vi "Power Supply Control Panel (No Objects).vi"(8 "error in (no error)":errorcluster) -> (0 "error out":errorcluster)   [LabVIEW 2012]
uses:
  Magnet status.ctl
  Oxford/PSSUBS.LLB/PSIO.ctl
  Oxford/BUSGEN.LLB/OxfordAddress.ctl
  Power Supply.lvclass
panel:
  in  "tada":string="Sound\\XP Sounds\\tada.wav"
  out "*ips120 (No Ob)":T4={"Field"=0.0, "Rate"=0.0, "Status"={"Sweeping"=FALSE, "Clamped"=FALSE, "Hold"=FALSE, "At Rest"=FALSE, "Quench"=FALSE, "Persistent Mode"=FALSE, "Switch Heater"=FALSE}, "ILM Shut Down?"=FALSE, "IO Info"={"Address"={"Com Port"=1, "ISOBUS Address"=2, "GPIB Address"=24, "Communication"=enum."ISOBUS"}, "Version"=enum."IPS"}, "IO Info (Level Meter)"={"Address"={"Com Port"=1, "ISOBUS Address"=5, "GPIB Address"=24, "Communication"=enum."ISOBUS"}, "ILM Name"="", "Display Channel"=[]}, "Training?"=FALSE, "Training Field and Speed Cluster"={"Training Field"=[0.0, 4.108, 5.78, 8.001], "Training Speed"=[0.0057, 0.0022833333333333334, 0.0011333333333333334, 0.0011333333333333334]}}
  in  "Cluster In":T4={"Field"=0.0, "Rate"=0.0, "Status"={"Sweeping"=FALSE, "Clamped"=FALSE, "Hold"=FALSE, "At Rest"=FALSE, "Quench"=FALSE, "Persistent Mode"=FALSE, "Switch Heater"=FALSE}, "ILM Shut Down?"=FALSE, "IO Info"={"Address"={"Com Port"=1, "ISOBUS Address"=2, "GPIB Address"=24, "Communication"=enum."ISOBUS"}, "Version"=enum."IPS"}, "IO Info (Level Meter)"={"Address"={"Com Port"=1, "ISOBUS Address"=5, "GPIB Address"=24, "Communication"=enum."ISOBUS"}, "ILM Name"="", "Display Channel"=[]}, "Training?"=FALSE, "Training Field and Speed Cluster"={"Training Field"=[0.0, 4.108, 5.78, 8.001], "Training Speed"=[0.0057, 0.0022833333333333334, 0.0011333333333333334, 0.0011333333333333334]}}
  out "Was at persistent?":bool
  in  "Return to persistent?":bool
  out "log counter":dbl
  out "Going to Field?":bool
  out "Current Field":dbl[unit]
  out "Update UI":bool
  out "Status":T1
  in  "Abort Field Sweep":bool
  out "done?":bool
  out "ILM Shut Down?":bool
  out "SH On":bool caption="Switch Heater"
  out "Persistent Mode":bool
  in  "SHcontrol":bool caption="Switch Heater"
  in  "gotopersistent":bool
  out "active":bool
  in  "Train\nMagnet":bool
  out "Busy":bool
  out "ready?":bool
  in  "rate":dbl[unit]=0.016666666666666666 caption="Rate" min=0.0 max=0.25
  in  "Goto":dbl[unit]
  in  "Clamp":bool
  in  "Check for Magnet":bool
  in  "Hold":bool
  in  "Goto Zero":bool
  in  "Goto Field":bool
  in  "endprgm":bool
  # "Magnet Control Panel"
  # "(at current field)"
  # "Off"
  # "On"
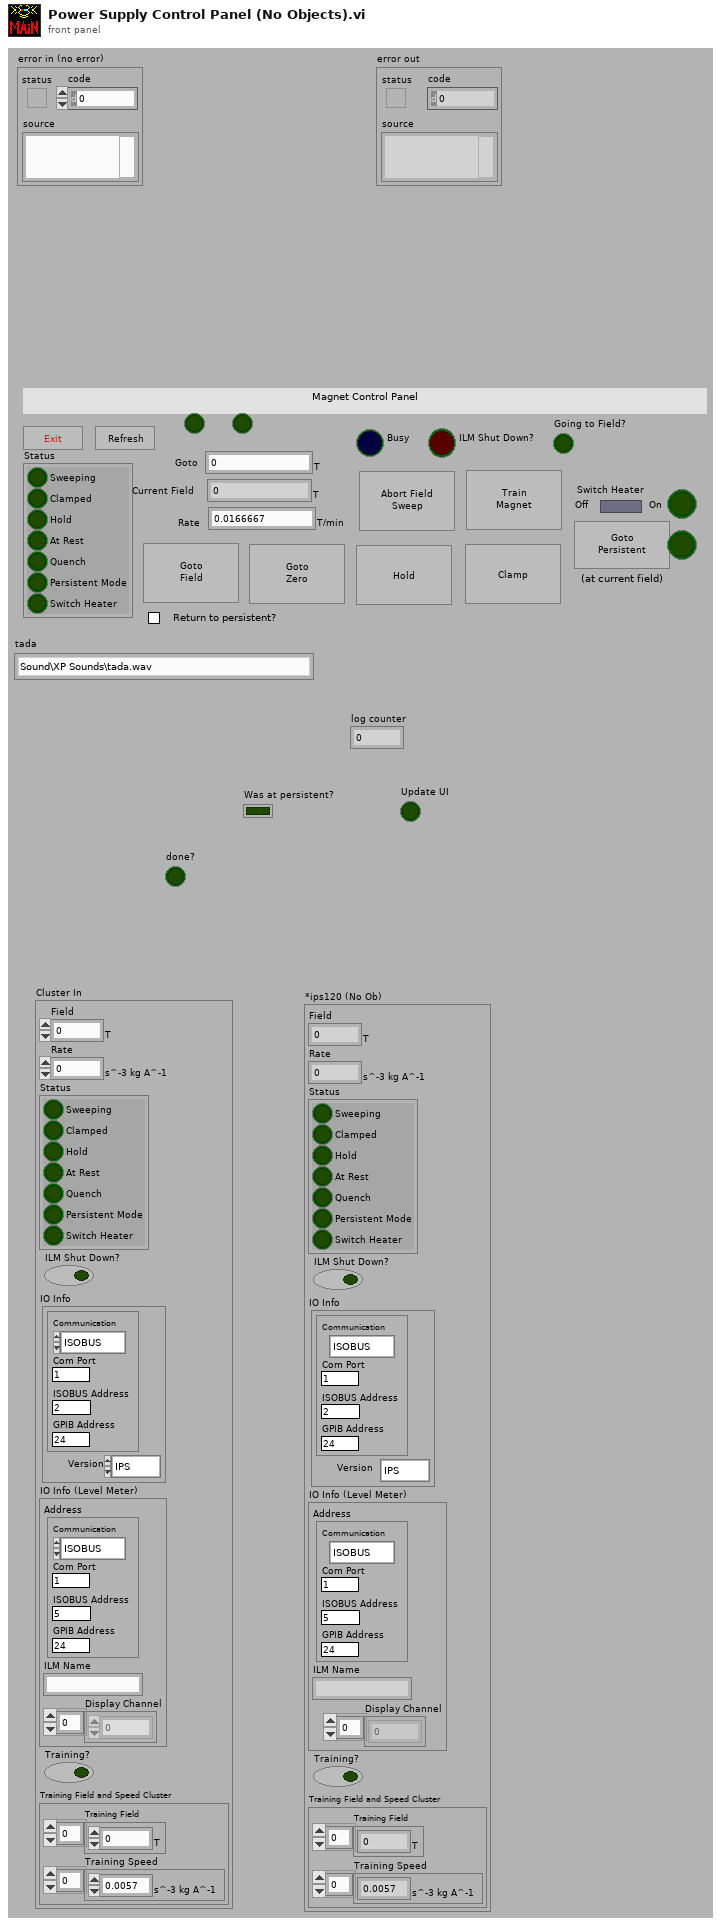
[diagram p1: front panel]
types:
  T1 = typedef "Power Supply.lvclass/Magnet status.ctl" = cluster{"Sweeping":bool, "Clamped":bool, "Hold":bool, "At Rest":bool, "Quench":bool, "Persistent Mode":bool, "Switch Heater":bool}
  T2 = typedef "PSIO.ctl" = cluster{"Address":T3, "Version":enum16{"PS", "IPS"}}
  T3 = typedef "OxfordAddress.ctl" = cluster{"Com Port":i32, "ISOBUS Address":i32, "GPIB Address":i16, "Communication":enum16{"RS232", "ISOBUS", "GPIB", "Gateway"}}
  T4 = cluster{"Field":dbl[unit], "Rate":dbl[unit], "Status":T1, "ILM Shut Down?":bool, "IO Info":T2, "IO Info (Level Meter)":cluster{"Address":T3, "ILM Name":string, "Display Channel":i32[]}, "Training?":bool, "Training Field and Speed Cluster":cluster{"Training Field":dbl[unit][], "Training Speed":dbl[unit][]}}
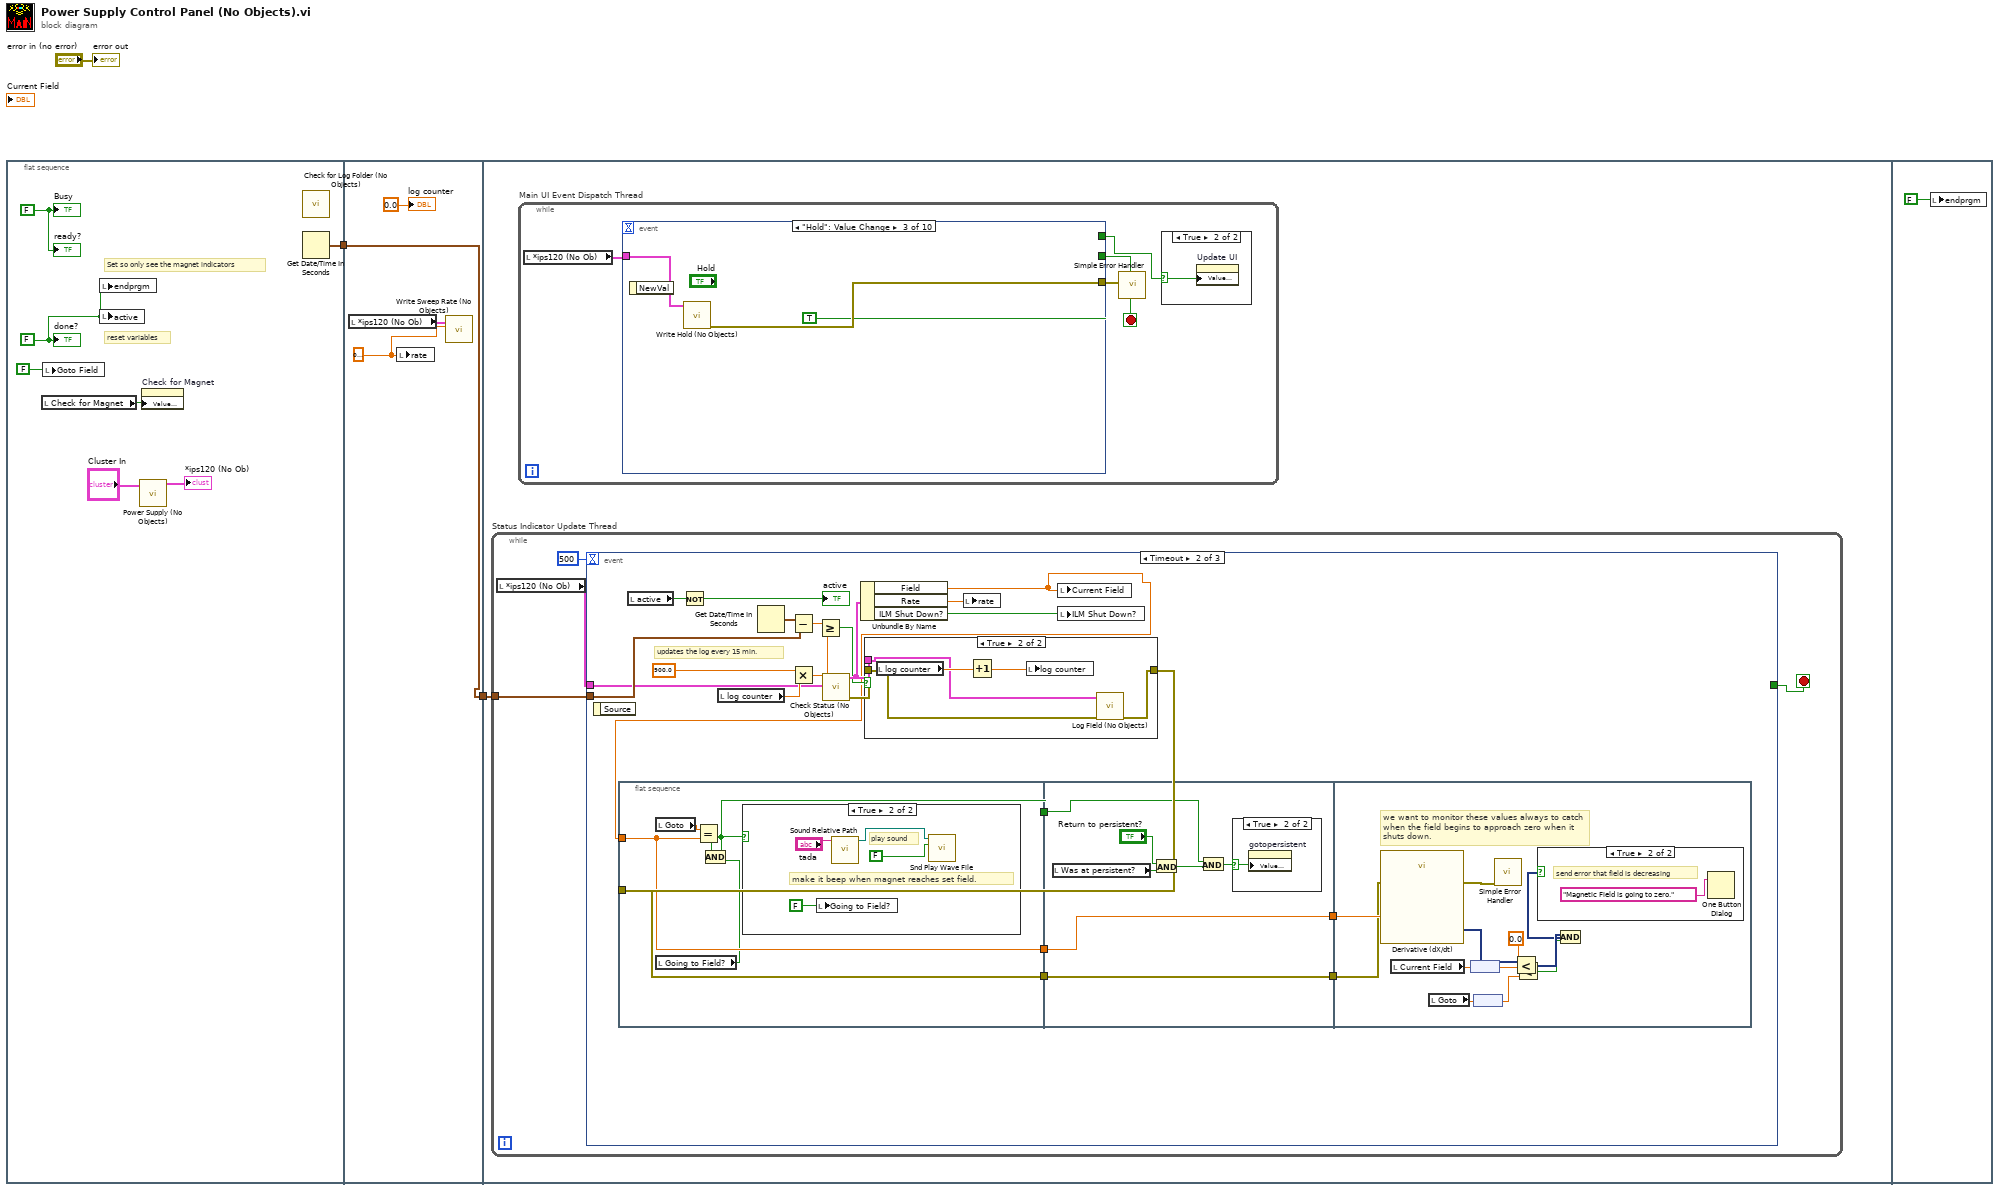
[diagram p0: block diagram]
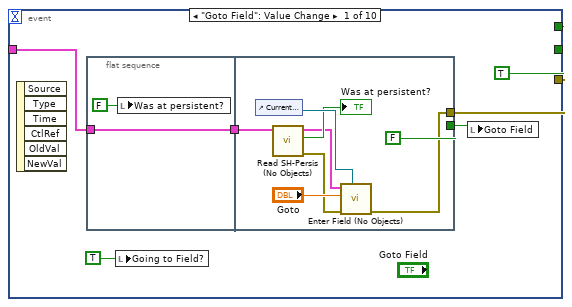
[diagram p3: hidden frame]
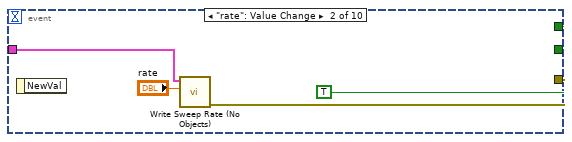
[diagram p4: hidden frame]
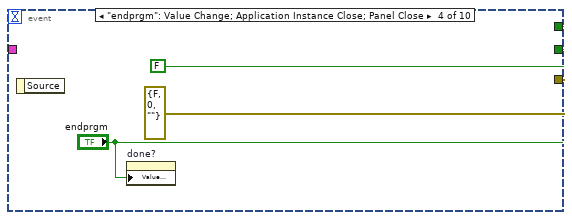
[diagram p5: hidden frame]
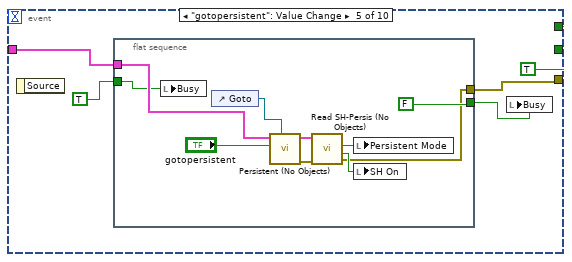
[diagram p6: hidden frame]
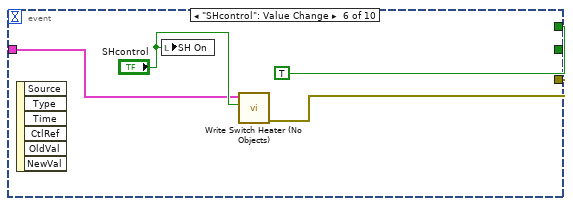
[diagram p7: hidden frame]
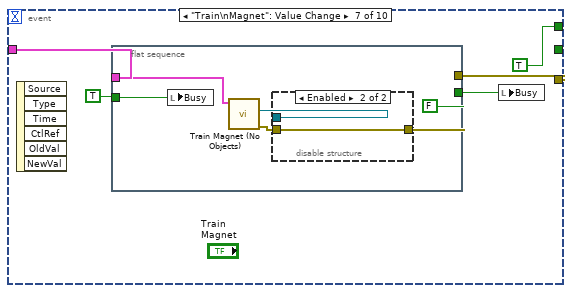
[diagram p8: hidden frame]
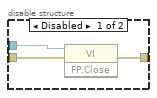
[diagram p9: hidden frame]
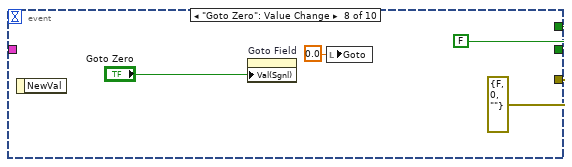
[diagram p10: hidden frame]
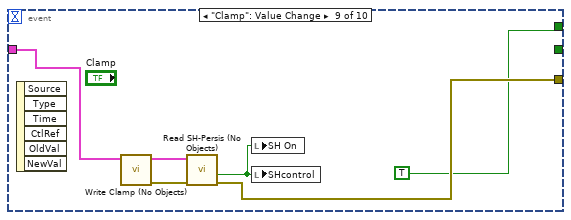
[diagram p11: hidden frame]
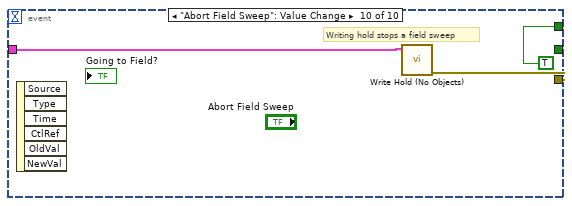
[diagram p12: hidden frame]
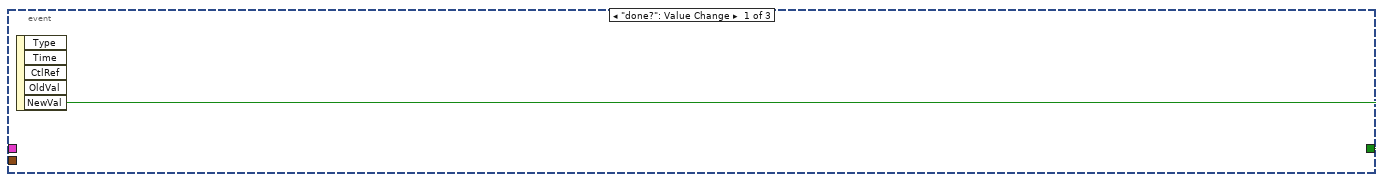
[diagram p13: hidden frame]
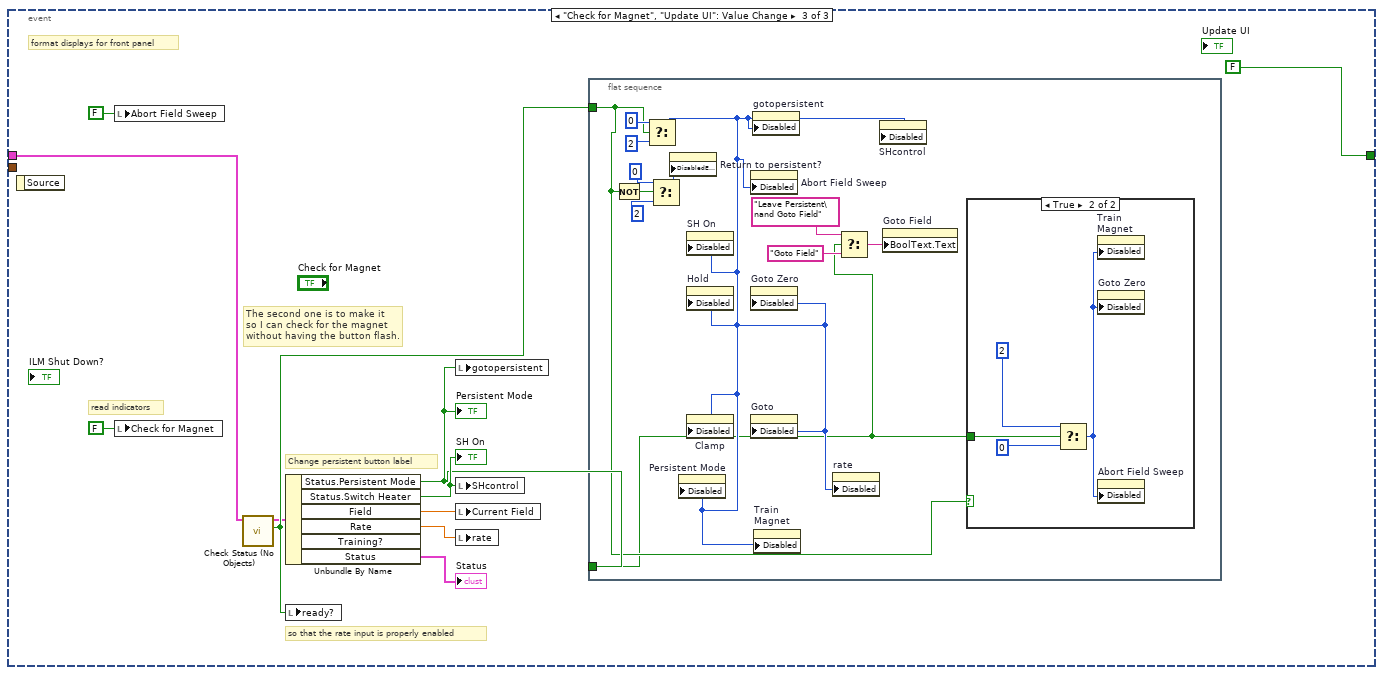
[diagram p18: hidden frame]
diagram:
  n1 = flat-sequence {
    tunnel: [w6] -> w2
    tunnel: w2 -> [w11]
    tunnel: [w11] -> w1
    tunnel: w1 -> [w15]
    frame #0 {
      w10 = FALSE
      w8 = FALSE
      # "Set so only see the magnet indicators"
      # "reset variables"
      n2 = local read "Check for Magnet"() -> (w9:bool)
      n3 = local write "Goto Field"(FALSE ("active")) -> ()
      n4 = local write "endprgm"(w8) -> ()
      n5 = local write "active"(w8) -> ()
      n6 = call "Power Supply (No Objects).vi"("Cluster In"="Cluster In") -> ("Cluster Out"=→"*ips120 (No Ob)":T4)  [unwired: 9 in, 1 out]
      n7 = property on="Check for Magnet" class="Bool (strict)"("Value (Signaling)"=w9) -> ()  [unwired: 2 in, 2 out]
      n8 = call "Check for Log Folder (No Objects).vi"() -> ()  [unwired: 1 in]
      n9 = Get Date/Time In Seconds() -> (seconds since 1Jan1904=w6:timestamp)
      "ready?" <- w10
      "Busy" <- w10
      "done?" <- w8
    }
    frame #1 {
      w12 = dbl[unit] 0.016666666666666666 ("rate")
      n10 = local read "*ips120 (No Ob)"() -> (w13:T4)
      n11 = local write "rate"(w12) -> ()
      n12 = call "Write Sweep Rate (No Objects).vi"("rate"=w12, "Cluster In"=w13) -> ()  [unwired: 8 in, 2 out]
      "log counter" <- 0.0 ("log counter")
    }
    frame #2 {
      n13 = while "Status Indicator Update Thread" {
        tunnel: w15 -> [w96]
        stop <- w94 stop-if-true
        n14 = local read "*ips120 (No Ob)"() -> (w95:T4)
        n15 = event shown="[1] Timeout" {
          selector: _ -> [_ _ _]
          dyn-events: _ -> [_ _ _]
          timeout: 500 -> [_ _ _]
          tunnel: [w98 _ FALSE] -> w94
          tunnel: w95 -> [_ w101 w158]
          tunnel: w96 -> [_ w117 _]
          event "done?": Value Change {
            n16 = event-data() -> ("NewVal"=w98:bool)  [unwired: 5 out]
          }
          event Timeout {
            # "updates the log every 15 min."
            n17 = event-data() -> ()  [unwired: 2 out]
            n18 = flat-sequence {
              tunnel: w100 -> [w125]
              tunnel: w99 -> [w123]
              tunnel: [w123] -> w106
              tunnel: [w125] -> w105
              tunnel: [w120] -> w104
              tunnel: w106 -> [w136]
              tunnel: [w136] -> w103
              tunnel: w105 -> [w135]
              tunnel: [w135] -> w102
              tunnel: w104 -> [w133]
              tunnel: w103 -> [w149]
              tunnel: w102 -> [w148]
              frame #0 {
                n19 = local read "Goto"() -> (w124:dbl[unit])
                n20 = local read "Going to Field?"() -> (w121:bool)
                n21 = Equal?(x=w124, y=w123) -> (x = y?=w122:bool)
                n22 = And(x=w122, y=w121) -> (x .and. y?=w120:bool)
                n23 = case shown="True" w120 {
                  frame False {
                  }
                  frame True {
                    # "make it beep when magnet reaches set field."
                    # "play sound"
                    n24 = local write "Going to Field?"(FALSE ("Going to Field?")) -> ()
                    n25 = call "Sound Relative Path.vi"("Sound"="tada") -> ("Relative Path"=w128:path)  [unwired: 10 in]
                    n26 = call <vilib>:"Snd Play Wave File.vi"("wait until finish (T)"=FALSE, "wave file path"=w128) -> ()  [unwired: 1 in, 9 out]
                  }
                }
              }
              frame #1 {
                n27 = local read "Was at persistent?"() -> (w132:bool)
                n28 = And(x="Return to persistent?", y=w132) -> (x .and. y?=w130:bool)
                n29 = And(x=w133, y=w130) -> (x .and. y?=w134:bool)
                n30 = case shown="True" w134 {
                  selector: w134 -> [_ w137]
                  frame False {
                  }
                  frame True {
                    n31 = property on="gotopersistent" class="Bool (strict)"("Value (Signaling)"=w137) -> ()  [unwired: 2 in, 2 out]
                  }
                }
              }
              frame #2 {
                # "we want to monitor these values always to catch\nwhen the field begins to approach zero when it\nshuts down."
                n32 = call "Derivative (dX/dt)"("error in (no error)"=w148, "Signals"=w149) -> ("error out"=w143:errorcluster, "Result"=w147:dynamicdata)  [unwired: 4 out]
                n33 = local read "Current Field"() -> (w139:dbl[unit])
                n34 = local read "Goto"() -> (w141:dbl[unit])
                n35 = node(w139) -> (w138:dbl)
                n36 = node(w141) -> (w140:dbl)
                n37 = call <vilib>:"Simple Error Handler.vi"("error in (no error)"=w143) -> ()  [unwired: 4 in, 5 out]
                n38 = Less?(x=w147, y=0.0) -> (x < y?=w145:dynamicdata)
                n39 = Less?(x=w138, y=w140) -> (x < y?=w142:bool)
                n40 = And(x=w145, y=w142) -> (x .and. y?=w144:dynamicdata)
                n41 = case shown="True" w144 {
                  frame False {
                  }
                  frame True {
                    # "send error that field is decreasing"
                    n42 = One Button Dialog(message="Magnetic Field is going to zero.") -> ()  [unwired: 1 in, 1 out]
                  }
                }
              }
            }
            n43 = local read "active"() -> (w119:bool)
            n44 = Not(x=w119) -> (.not. x?=→"active":bool)
            n45 = local read "log counter"() -> (w109:dbl)
            n46 = Get Date/Time In Seconds() -> (seconds since 1Jan1904=w112:timestamp)
            n47 = Subtract(x=w112, y=w117) -> (x-y=w107:dbl)
            n48 = Multiply(x=900.0 ("millisecond multiple"), y=w109) -> (x*y=w108:dbl)
            n49 = Greater Or Equal?(x=w107, y=w108) -> (x >= y?=w113:bool)
            n50 = call "Check Status (No Objects).vi"("Cluster In"=w101) -> ("error out"=w114:errorcluster, "Cluster Out"=w115:T4)  [unwired: 7 in, 2 out]
            n51 = Unbundle By Name(w115) -> ("Field"=w99:dbl[unit], "Rate"=w111:dbl[unit], "ILM Shut Down?"=w116:bool)
            n52 = case shown="True" w113 {
              tunnel: [w151 w156] -> w100
              tunnel: w115 -> [_ w153]
              tunnel: w114 -> [w151 w152]
              frame False {
              }
              frame True {
                n53 = local read "log counter"() -> (w155:dbl)
                n54 = Increment(x=w155) -> (x+1=w154:dbl)
                n55 = local write "log counter"(w154) -> ()
                n56 = call "Log Field (No Objects).vi"("error in (no error)"=w152, "Cluster In"=w153) -> ("error out"=w156:errorcluster)  [unwired: 8 in, 1 out]
              }
            }
            n57 = local write "rate"(w111) -> ()
            n58 = local write "Current Field"(w99) -> ()
            n59 = local write "ILM Shut Down?"(w116) -> ()
          }
          event "Check for Magnet", "Update UI": Value Change {
            # "format displays for front panel"
            # "read indicators"
            # "so that the rate input is properly enabled"
            # "Change persistent button label"
            # "The second one is to make it\nso I can check for the magnet\nwithout having the button flash."
            n60 = event-data() -> ()  [unwired: 2 out]
            n61 = local write "Abort Field Sweep"(FALSE ("Abort Field Sweep")) -> ()
            n62 = local write "Check for Magnet"(FALSE) -> ()
            n63 = call "Check Status (No Objects).vi"("Cluster In"=w158) -> ("Ready?"=w166:bool, "Cluster Out"=w164:T4)  [unwired: 7 in, 2 out]
            n64 = Unbundle By Name(w164) -> ("Status.Persistent Mode"=w161:bool, "Status.Switch Heater"=w165:bool, "Field"=w162:dbl[unit], "Rate"=w159:dbl[unit], "Status"=→"Status":T1)  [unwired: 1 out]
            "Persistent Mode" <- w161
            "SH On" <- w165
            n65 = local write "ready?"(w166) -> ()
            n66 = local write "gotopersistent"(w161) -> ()
            n67 = local write "SHcontrol"(w165) -> ()
            n68 = local write "Current Field"(w162) -> ()
            n69 = local write "rate"(w159) -> ()
            n70 = flat-sequence {
              tunnel: w161 -> [w168]
              tunnel: w166 -> [w174]
              frame #0 {
                n71 = Not(x=w174) -> (.not. x?=w173:bool)
                n72 = Select(t=0, s=w174, f=2) -> (s? t:f=w177:i32)
                n73 = Select(t=0, s=w173, f=2) -> (s? t:f=w172:i32)
                n74 = property on="Return to persistent?" class="Bool (strict)"("DisabledEnum"=w172) -> ()  [unwired: 2 in, 2 out]
                n75 = property on="Persistent Mode" class="Bool (strict)"("Disabled"=w177) -> ()  [unwired: 2 in, 2 out]
                n76 = property on="SH On" class="Bool (strict)"("Disabled"=w177) -> ()  [unwired: 2 in, 2 out]
                n77 = property on="Hold" class="Bool"("Disabled"=w177) -> ()  [unwired: 2 in, 2 out]
                n78 = property on="Clamp" class="Bool"("Disabled"=w177) -> ()  [unwired: 2 in, 2 out]
                n79 = property on="Abort Field Sweep" class="Bool (strict)"("Disabled"=w177) -> ()  [unwired: 2 in, 2 out]
                n80 = property on="Goto Zero" class="Bool"("Disabled"=w177) -> ()  [unwired: 2 in, 2 out]
                n81 = property on="Goto" class="DigNum (strict)"("Disabled"=w177) -> ()  [unwired: 2 in, 2 out]
                n82 = property on="gotopersistent" class="Bool (strict)"("Disabled"=w177) -> ()  [unwired: 2 in, 2 out]
                n83 = property on="Train\nMagnet" class="Bool"("Disabled"=w177) -> ()  [unwired: 2 in, 2 out]
                n84 = property on="rate" class="DigNum (strict)"("Disabled"=w177) -> ()  [unwired: 2 in, 2 out]
                n85 = Select(t="Leave Persistent\nand Goto Field", s=w168, f="Goto Field") -> (s? t:f=w170:string)
                n86 = property on="SHcontrol" class="Bool (strict)"("Disabled"=w177) -> ()  [unwired: 2 in, 2 out]
                n87 = property on="Goto Field" class="Bool (strict)"("BoolText.Text"=w170) -> ()  [unwired: 2 in, 2 out]
                n88 = case shown="True" w174 {
                  tunnel: w168 -> [_ w181]
                  frame False {
                  }
                  frame True {
                    n89 = Select(t=2, s=w181, f=0) -> (s? t:f=w180:i32)
                    n90 = property on="Train\nMagnet" class="Bool"("Disabled"=w180) -> ()  [unwired: 2 in, 2 out]
                    n91 = property on="Goto Zero" class="Bool"("Disabled"=w180) -> ()  [unwired: 2 in, 2 out]
                    n92 = property on="Abort Field Sweep" class="Bool (strict)"("Disabled"=w180) -> ()  [unwired: 2 in, 2 out]
                  }
                }
              }
            }
          }
        }
      }
      n93 = while "Main UI Event Dispatch Thread" {
        stop <- w18 stop-if-true
        n94 = local read "*ips120 (No Ob)"() -> (w16:T4)
        n95 = event shown="[2] \"Hold\": Value Change" {
          selector: _ -> [_ _ _ _ _ _ _ _ _ _]
          dyn-events: _ -> [_ _ _ _ _ _ _ _ _ _]
          timeout: _ -> [_ _ _ _ _ _ _ _ _ _]
          tunnel: [_ _ _ "endprgm" _ _ _ _ _ _] -> w18
          tunnel: w16 -> [w26 w39 w42 _ w48 w64 w70 _ w85 w92]
          tunnel: [w21 w37 w43 errorcluster {"status"=FALSE, "code"=0, "source"=""} ("error out") w51 w62 w69 errorcluster {"status"=FALSE, "code"=0, "source"=""} ("error out") w88 w93] -> w19
          tunnel: [TRUE TRUE TRUE FALSE TRUE TRUE TRUE FALSE TRUE TRUE] -> w17
          event "Goto Field": Value Change {
            n96 = event-data() -> ()  [unwired: 7 out]
            n97 = flat-sequence {
              tunnel: w26 -> [w28]
              tunnel: [w28] -> w23
              tunnel: [FALSE ("Goto Field")] -> w25
              tunnel: [w29] -> w21
              tunnel: w23 -> [w31]
              frame #0 {
                n98 = local write "Was at persistent?"(FALSE ("Was at persistent?")) -> ()
              }
              frame #1 {
                n99 = control-ref of="Current Field"() -> (w35:refnum<vi>)
                n100 = call "Read SH-Persis (No Objects).vi"("Cluster In"=w31) -> ("error out"=w33:errorcluster, "pers?"=→"Was at persistent?":bool, "Cluster Out"=w30:T4)  [unwired: 5 in, 3 out]
                n101 = call "Enter Field (No Objects).vi"("Field monitor"=w35, "error in (no error)"=w33, "Target field"="Goto", "Cluster In"=w30) -> ("error out"=w29:errorcluster)  [unwired: 6 in, 1 out]
              }
            }
            n102 = local write "Going to Field?"(TRUE ("Going to Field?")) -> ()
            n103 = local write "Goto Field"(w25) -> ()
          }
          event "rate": Value Change {
            n104 = event-data() -> ()  [unwired: 2 out]
            n105 = call "Write Sweep Rate (No Objects).vi"("rate"="rate", "Cluster In"=w39) -> ("error out"=w37:errorcluster)  [unwired: 8 in, 1 out]
          }
          event "Hold": Value Change {
            n106 = event-data() -> ()  [unwired: 2 out]
            n107 = call "Write Hold (No Objects).vi"("Cluster In"=w42) -> ("error out"=w43:errorcluster)  [unwired: 9 in, 1 out]
          }
          event "endprgm": Value Change; Application Instance Close; Panel Close {
            n108 = event-data() -> ()  [unwired: 2 out]
            n109 = property on="done?" class="Bool (strict)"("Value (Signaling)"="endprgm") -> ()  [unwired: 2 in, 2 out]
          }
          event "gotopersistent": Value Change {
            n110 = event-data() -> ()  [unwired: 2 out]
            n111 = flat-sequence {
              tunnel: w48 -> [w55]
              tunnel: [w53] -> w51
              tunnel: TRUE -> [w52]
              tunnel: [FALSE] -> w49
              frame #0 {
                n112 = local write "Busy"(w52) -> ()
                n113 = control-ref of="Goto"() -> (w60:refnum<vi>)
                n114 = call "Persistent (No Objects).vi"("Field monitor ref"=w60, "Go to persistent mode?"="gotopersistent", "Cluster In"=w55) -> ("error out"=w61:errorcluster, "Cluster Out"=w54:T4)  [unwired: 7 in]
                n115 = call "Read SH-Persis (No Objects).vi"("error in (no error)"=w61, "Cluster In"=w54) -> ("error out"=w53:errorcluster, "SHon?"=w57:bool, "pers?"=w58:bool)  [unwired: 4 in, 3 out]
                n116 = local write "Persistent Mode"(w58) -> ()
                n117 = local write "SH On"(w57) -> ()
              }
            }
            n118 = local write "Busy"(w49) -> ()
          }
          event "SHcontrol": Value Change {
            n119 = event-data() -> ()  [unwired: 7 out]
            n120 = local write "SH On"("SHcontrol") -> ()
            n121 = call "Write Switch Heater (No Objects).vi"("Turn SH On?"="SHcontrol", "Cluster In"=w64) -> ("error out"=w62:errorcluster)  [unwired: 8 in, 1 out]
          }
          event "Train\nMagnet": Value Change {
            n122 = event-data() -> ()  [unwired: 7 out]
            n123 = flat-sequence {
              tunnel: w70 -> [w71]
              tunnel: [w72] -> w69
              tunnel: [FALSE] -> w68
              tunnel: TRUE -> [w75]
              frame #0 {
                n124 = local write "Busy"(w75) -> ()
                n125 = call "Train Magnet (No Objects).vi"("Cluster In"=w71) -> ("error out"=w73:errorcluster, "This VI"=w74:refnum<vi>)  [unwired: 8 in, 1 out]
                n126 = disable-structure shown="Enabled" {
                  disable-tunnel: w74 -> [w79 _]
                  disable-tunnel: w73 -> [w78 w80]
                  disable-tunnel: [w77 w80] -> w72
                  frame Disabled {
                    n127 = invoke class="VI" method="FP.Close"(reference=w79, error in=w78) -> (error out=w77:errorcluster)  [unwired: 1 in, 2 out]
                  }
                  frame Enabled {
                  }
                }
              }
            }
            n128 = local write "Busy"(w68) -> ()
          }
          event "Goto Zero": Value Change {
            n129 = event-data() -> ()  [unwired: 2 out]
            n130 = property on="Goto Field" class="Bool (strict)"("Val(Sgnl)"="Goto Zero") -> ()  [unwired: 2 in, 2 out]
            n131 = local write "Goto"(dbl[unit] 0.0 ("Goto")) -> ()
          }
          event "Clamp": Value Change {
            n132 = event-data() -> ()  [unwired: 7 out]
            n133 = call "Write Clamp (No Objects).vi"("Cluster In"=w85) -> ("error out"=w90:errorcluster, "Cluster Out"=w87:T4)  [unwired: 9 in]
            n134 = call "Read SH-Persis (No Objects).vi"("error in (no error)"=w90, "Cluster In"=w87) -> ("error out"=w88:errorcluster, "SHon?"=w89:bool)  [unwired: 4 in, 4 out]
            n135 = local write "SH On"(w89) -> ()
            n136 = local write "SHcontrol"(w89) -> ()
          }
          event "Abort Field Sweep": Value Change {
            # "Writing hold stops a field sweep"
            n137 = event-data() -> ()  [unwired: 7 out]
            n138 = call "Write Hold (No Objects).vi"("Cluster In"=w92) -> ("error out"=w93:errorcluster)  [unwired: 9 in, 1 out]
          }
        }
        n139 = call <vilib>:"Simple Error Handler.vi"("error in (no error)"=w19) -> ()  [unwired: 4 in, 5 out]
        n140 = case shown="True" w17 {
          selector: w17 -> [_ w20]
          frame False {
          }
          frame True {
            n141 = property on="Update UI" class="Bool (strict)"("Value (Signaling)"=w20) -> ()  [unwired: 2 in, 2 out]
          }
        }
      }
    }
    frame #3 {
      n142 = local write "endprgm"(FALSE) -> ()
    }
  }
  "error out" <- "error in (no error)"
